vi "Get Serial Settings.vi"(8 "error IO":errorcluster, 11 "Module Configuration in":refnum<class "Module Configuration.lvclass">) -> (0 "error IO Out":errorcluster, 2 "Serial Configuration":T1={"VISA"="", "Interface Type"=0, "Serial Interface"={"Baud Rate"=19200, "Data Bits "=8, "Parity"=enum."None", "Stop Bits"=0}, "Slave Address"=1} {"Interface Type" items=["GPIB"=1, "VXI"=2, "GPIB-VXI"=3, "Serial"=4, "PXI"=5, "TCPIP"=6, "USB"=7, "FireWire"=9, "Invalid"=0]; "Serial Interface"."Stop Bits" items=["1.0", "1.5", "2.0"]; "Serial Interface"."Baud Rate" items=["1200"=1200, "2400"=2400, "4800"=4800, "9600"=9600, "19200"=19200, "38400"=38400, "57600"=57600, "115200"=115200]; "Slave Address" format="%.0x"}, 3 "Module Configuration out":refnum<class "Module Configuration.lvclass">)   [LabVIEW 2020, in "Plugin.lvlib" / "Plugin_UI.lvclass"]
doc: "Reads the Hardware Configuration"
uses:
  Plugin_UI.lvclass
  Serial Configuration.ctl
  builds/Libraries/Shared GUI Library.lvlibp/Shared GUI Library/Instrument Settings/Interface/Interface Type.ctl
  builds/Libraries/Shared GUI Library.lvlibp/Shared GUI Library/Instrument Settings/Interface/Serial Interafce.ctl
  builds/Libraries/LabSys Framework.lvlibp/Configuration Storage/Module Configuration/Module Configuration.lvclass
  builds/Libraries/Shared GUI Library.lvlibp
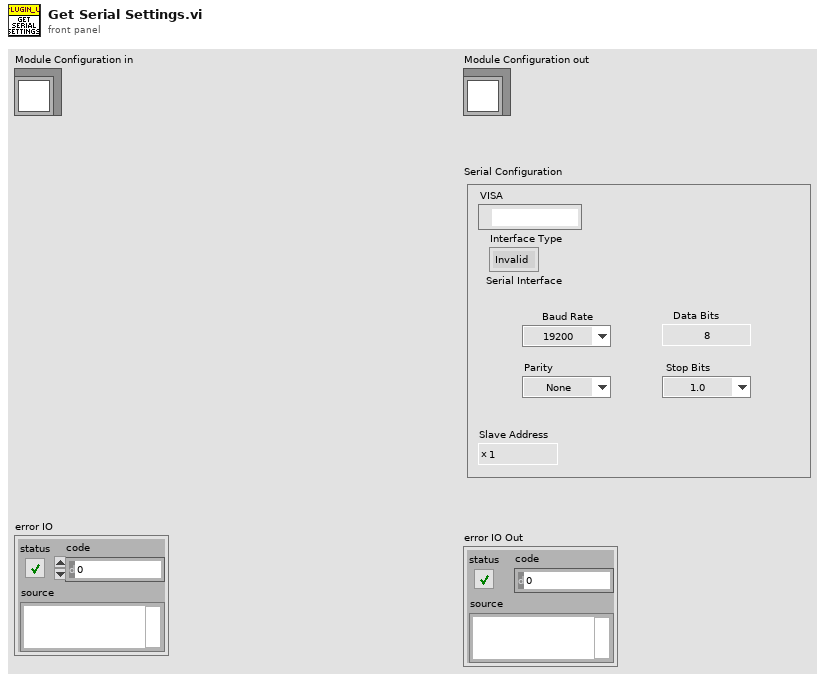
[diagram p1: front panel]
types:
  T1 = typedef "Plugin.lvlib/Plugin_UI.lvclass/Serial Configuration.ctl" = cluster{"VISA":refnum<visa-resource-name>, "Interface Type":T2, "Serial Interface":T3, "Slave Address":u8}
  T2 = typedef "Shared GUI Library.lvlibp/Interface Type.ctl" = u16
  T3 = typedef "Shared GUI Library.lvlibp/Serial Interafce.ctl" = cluster{"Baud Rate":u32, "Data Bits ":u16, "Parity":enum16{"None", "Odd", "Even"}, "Stop Bits":u16}
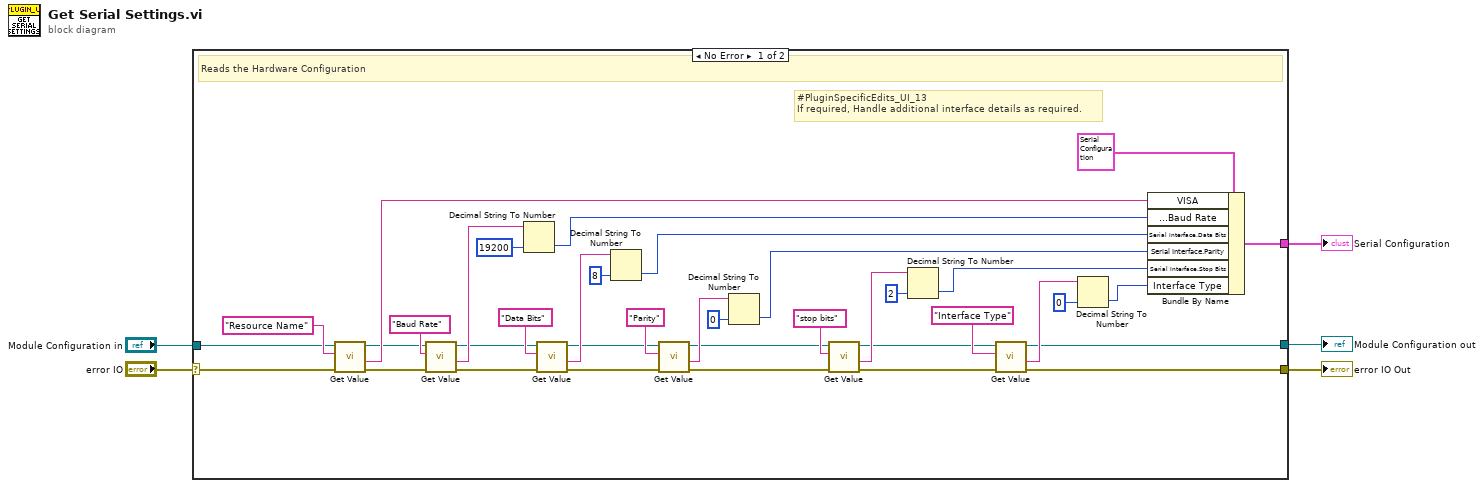
[diagram p0: block diagram]
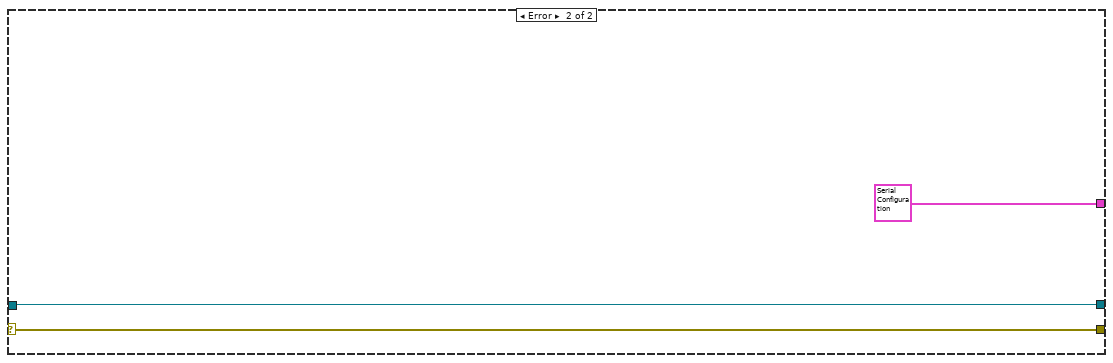
[diagram p2: hidden frame]
diagram:
  n1 = case shown="No Error" "error IO" {
    selector: "error IO" -> [w11 w46]
    tunnel: [w8 w46] -> w1
    tunnel: "Module Configuration in" -> [w10 w45]
    tunnel: [w7 w45] -> w2
    tunnel: [w9 T1 {"VISA"="", "Interface Type"=0, "Serial Interface"={"Baud Rate"=19200, "Data Bits "=8, "Parity"=enum."None", "Stop Bits"=0}, "Slave Address"=1} ("Serial Configuration")] -> w3
    frame No Error {
      # "#PluginSpecificEdits_UI_13\nIf required, Handle additional interface details as required."
      # "Reads the Hardware Configuration"
      n2 = call "Get Value.vi"("error in (no error)"=w11, "Key"="Resource Name", "Module Configuration in"=w10) -> ("error out"=w43:errorcluster, "Value"=w35:string, "Module Configuration out"=w26:refnum<class "Module Configuration.lvclass">)  [unwired: 6 in]
      n3 = call "Get Value.vi"("error in (no error)"=w43, "Key"="Baud Rate", "Module Configuration in"=w26) -> ("error out"=w42:errorcluster, "Value"=w36:string, "Module Configuration out"=w27:refnum<class "Module Configuration.lvclass">)  [unwired: 6 in]
      n4 = Decimal String To Number(string=w36, default (0L)=u32 19200 ("default (0 I32)")) -> (number=w25:u32)  [unwired: 1 in, 1 out]
      n5 = call "Get Value.vi"("error in (no error)"=w42, "Key"="Data Bits", "Module Configuration in"=w27) -> ("error out"=w41:errorcluster, "Value"=w37:string, "Module Configuration out"=w28:refnum<class "Module Configuration.lvclass">)  [unwired: 6 in]
      n6 = Decimal String To Number(string=w37, default (0L)=u16 8 ("default (0 I32)")) -> (number=w22:u16)  [unwired: 1 in, 1 out]
      n7 = call "Get Value.vi"("error in (no error)"=w41, "Key"="Parity", "Module Configuration in"=w28) -> ("error out"=w40:errorcluster, "Value"=w38:string, "Module Configuration out"=w29:refnum<class "Module Configuration.lvclass">)  [unwired: 6 in]
      n8 = Decimal String To Number(string=w38, default (0L)=u16 0 ("default (0 I32)")) -> (number=w23:u16)  [unwired: 1 in, 1 out]
      n9 = call "Get Value.vi"("error in (no error)"=w40, "Key"="stop bits", "Module Configuration in"=w29) -> ("error out"=w14:errorcluster, "Value"=w39:string, "Module Configuration out"=w15:refnum<class "Module Configuration.lvclass">)  [unwired: 6 in]
      n10 = Decimal String To Number(string=w39, default (0L)=u16 2 ("default (0 I32)")) -> (number=w24:u16)  [unwired: 1 in, 1 out]
      n11 = call "Get Value.vi"("error in (no error)"=w14, "Key"="Interface Type", "Module Configuration in"=w15) -> ("error out"=w8:errorcluster, "Value"=w13:string, "Module Configuration out"=w7:refnum<class "Module Configuration.lvclass">)  [unwired: 6 in]
      n12 = Decimal String To Number(string=w13, default (0L)=u16 0 ("default (0 I32)")) -> (number=w12:u16)  [unwired: 1 in, 1 out]
      n13 = Bundle By Name(cluster=T1 {"VISA"="", "Interface Type"=0, "Serial Interface"={"Baud Rate"=19200, "Data Bits "=8, "Parity"=enum."None", "Stop Bits"=0}, "Slave Address"=1} ("Serial Configuration"), "VISA"=w35, "Serial Interface.Baud Rate"=w25, "Serial Interface.Data Bits"=w22, "Serial Interface.Parity"=w23, "Serial Interface.Stop Bits"=w24, "Interface Type"=w12) -> (w9:T1)
    }
    frame Error {
    }
  }
  "Serial Configuration" <- w3
  "Module Configuration out" <- w2
  "error IO Out" <- w1
